vi "tsdb_get_flexray_db_count.vi"(8 "error in (no error)":errorcluster caption="错误输入（无错误）", 11 "path in":path) -> (0 "error out":errorcluster caption="错误输出", 1 "ACount out":i32, 2 "function return":i32, 3 "path out":path)   [LabVIEW 2014]
doc: "Function introduction: Get the total number of loaded flexray databases\nCall location\nInput parameter ACount: Return database count\nReturn value==0: Successful execution\nOther values: Query error code"
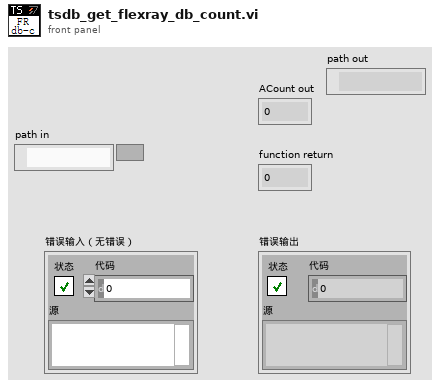
[diagram p1: front panel]
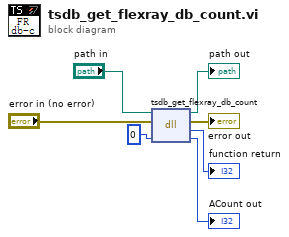
[diagram p0: block diagram]
diagram:
  n1 = dll-call lib="D:/Work/LabVIEW Code/TSMaster Labview SDK/LabVIEW/LabVIEW-TSMasterAPI_CLN/TSMasterAPI_LabVIEW-2024-10-08 14-20-13/Not_organized_vi/TSMaster.*" fn="tsdb_get_flexray_db_count"(path in="path in", error in="error in (no error)", "ACount"=0) -> (path out=→"path out":path, error out=→"error out":errorcluster, "返回类型"=→"function return":i32, "ACount"=→"ACount out":i32)  [unwired: 1 in]
